vi "Save Report.vi"(2 "error in (no error)":errorcluster, 3 "Report Ref In":T1) -> (0 "error out":errorcluster, 1 "Report Ref Out":T1)   [LabVIEW 2013, in "XCel Report Engine.lvlib"]
doc: "Saves the current workbook to the output path specified by New Report.vi without closing the report session.\n\nThe report remains open and Report Ref can be used by subsequent report operations. If the output file already exists, it is overwritten.\n\nUse Close Report.vi when report generation is complete to release the session and its associated resources."
uses:
  XCel Report Engine.lvlib
  C:/Users/m.santucci/Documents/ChatGPT/LV_REPORT_ENGINE/LV/DotNet/XCelReportEngine.dll
  LV/DotNet/XCelReportEngine.dll
  Controls/Report Ref.ctl
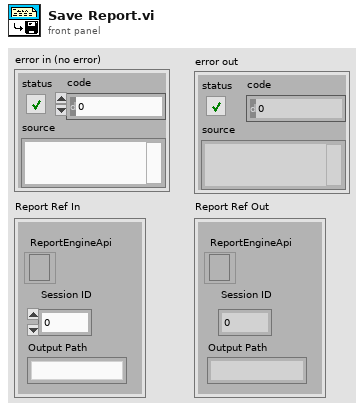
[diagram p1: front panel]
types:
  T1 = typedef "XCel Report Engine.lvlib/Report Ref.ctl" = cluster{"Session ID":i32, "Output Path":string, "ReportEngineApi":refnum<k24>}
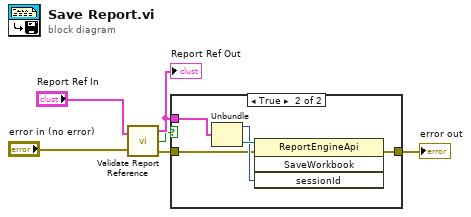
[diagram p0: block diagram]
diagram:
  n1 = call "Validate Report Reference.vi"("Report Ref In"="Report Ref In", "error in (no error)"="error in (no error)") -> ("Report Ref Out"=w4:T1, "Valid"=w1:bool, "error out"=w2:errorcluster)
  "Report Ref Out" <- w4
  n2 = case shown="True" w1 {
    tunnel: [w7 w11] -> w6
    tunnel: w4 -> [_ w9]
    tunnel: w2 -> [w7 w8]
    frame False {
    }
    frame True {
      n3 = Unbundle(w9) -> ("Session ID"=w10:i32, "ReportEngineApi"=w12:refnum<k24>)  [unwired: 1 out]
      n4 = invoke class="ReportEngineApi" method="SaveWorkbook"(reference=w12, error in=w8, "sessionId"=w10) -> (error out=w11:errorcluster)  [unwired: 1 in, 3 out]
    }
  }
  "error out" <- w6
